vi "Add N-complement Cursors.vi"(8 "Error In":errorcluster, 9 "Cursor Mode":T1(ring), 10 "Total Cursor Number":i32=2, 11 "CrsrList in":T2) -> (0 "Error Out":errorcluster, 3 "CrsrList out":T2)   [LabVIEW 2021, in "Graphs.lvlib"]
uses:
  Graphs.lvlib
  <vilib>/Utility/miscctls.llb/LVCursorListTypeDef.ctl
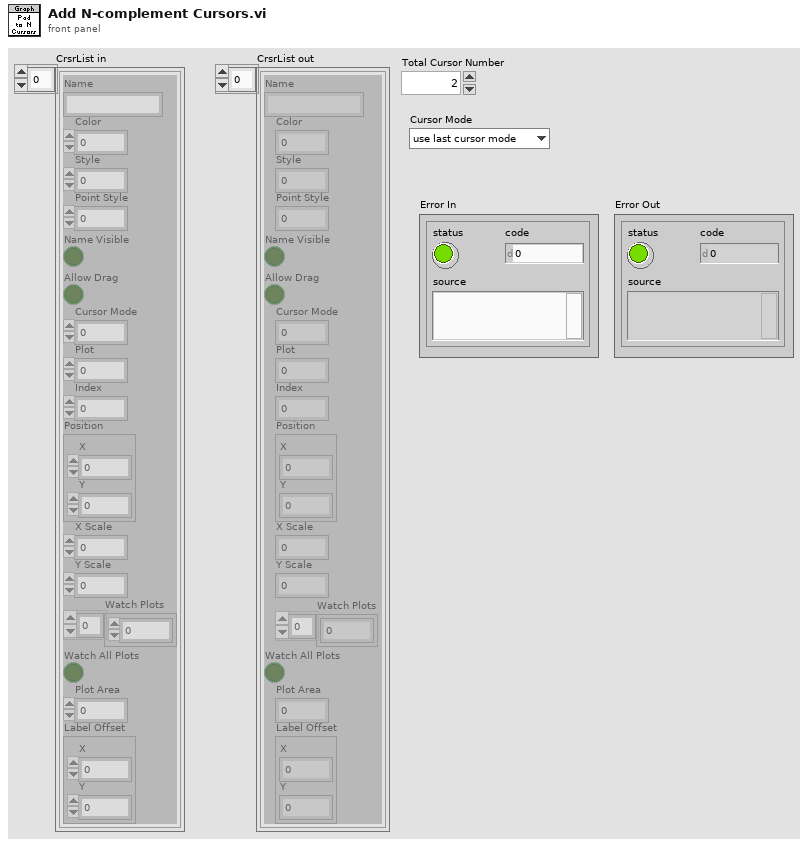
[diagram p1: front panel]
types:
  T1 = enum16{"use last cursor mode", "free", "single-plot", "multiplot"}
  T2 = typedef "LVCursorListTypeDef.ctl" = cluster{"Name":string, "Color":u32, "Style":u8, "Point Style":u8, "Name Visible":bool, "Allow Drag":bool, "Cursor Mode":u32, "Plot":i32, "Index":i32, "Position":cluster{"X":dbl, "Y":dbl}, "X Scale":u32, "Y Scale":u32, "Watch Plots":i32[], "Watch All Plots":bool, "Plot Area":i32, "Label Offset":cluster{"X":dbl, "Y":dbl}}[]
  T3 = cluster{"Name":string, "Color":u32, "Style":u8, "Point Style":u8, "Name Visible":bool, "Allow Drag":bool, "Cursor Mode":u32, "Plot":i32, "Index":i32, "Position":cluster{"X":dbl, "Y":dbl}, "X Scale":u32, "Y Scale":u32, "Watch Plots":i32[], "Watch All Plots":bool, "Plot Area":i32, "Label Offset":cluster{"X":dbl, "Y":dbl}}
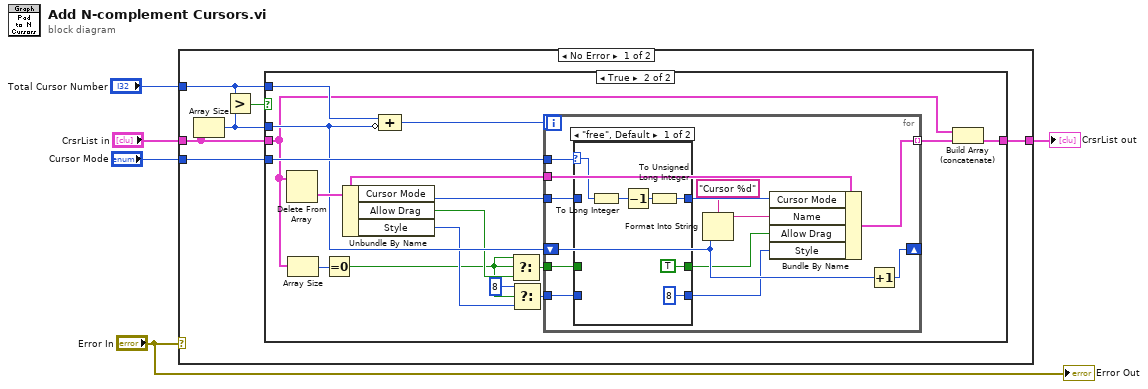
[diagram p0: block diagram]
diagram:
  n1 = case shown="No Error" "Error In" {
    tunnel: "CrsrList in" -> [w11 w51]
    tunnel: [w10 w51] -> w4
    tunnel: "Cursor Mode" -> [w9 _]
    tunnel: "Total Cursor Number" -> [w7 _]
    frame No Error {
      n2 = Array Size(array=w11) -> (size(s)=w8:i32)
      n3 = Greater?(x=w7, y=w8) -> (0:w6:bool)
      n4 = case shown="True" w6 {
        tunnel: w11 -> [w12 w13]
        tunnel: [w12 w14] -> w10
        tunnel: w8 -> [_ w23]
        tunnel: w9 -> [_ w27]
        tunnel: w7 -> [_ w24]
        frame False {
        }
        frame True {
          n5 = Delete From Array(array=w13) -> (deleted portion=w25:T3)  [unwired: 2 in, 1 out]
          n6 = Array Size(array=w13) -> (size(s)=w22:i32)
          n7 = Equal To 0?(x=w22) -> (x = 0?=w18:bool)
          n8 = Unbundle By Name(w25) -> ("Cursor Mode"=w26:u32, "Allow Drag"=w21:bool, "Style"=w19:u8)
          n9 = Compound Arithmetic op=ADD(w24, invert w23) -> (w28:i32)
          n10 = Select(t=w18, s=w18, f=w21) -> (s? t:f=w20:bool)
          n11 = Select(t=u8 8, s=w18, f=w19) -> (s? t:f=w16:u8)
          n12 = for {
            N: w28 -> [_]
            tunnel: w27 -> [w40]
            tunnel: w26 -> [w39]
            tunnel: w25 -> [w41]
            shift-right: [w37] -> _
            shift-left: w23 -> [w35]
            tunnel: w20 -> [w33]
            tunnel: w16 -> [w31]
            tunnel: [w29] -> w15 mode=indexing
            n13 = case shown="\"free\", Default" w40 {
              selector: w40 -> [w47 _]
              tunnel: w39 -> [_ w50]
              tunnel: [w44 w50] -> w38
              tunnel: w33 -> [_ w49]
              tunnel: [TRUE ("Allow Drag") w49] -> w32
              tunnel: w31 -> [_ w48]
              tunnel: [u8 8 ("Style") w48] -> w30
              frame "free", Default {
                n14 = To Long Integer(number=w47) -> (32bit integer=w45:i32)
                n15 = Decrement(x=w45) -> (x-1=w46:i32)
                n16 = To Unsigned Long Integer(number=w46) -> (unsigned 32bit integer=w44:u32)
              }
              frame "use last cursor mode" {
              }
            }
            n17 = Format Into String(format string="Cursor %d", w35) -> (resulting string=w36:string)  [unwired: 2 in, 1 out]
            n18 = Bundle By Name(cluster=w41, "Cursor Mode"=w38, "Name"=w36, "Allow Drag"=w32, "Style"=w30) -> (w29:T3)
            n19 = Increment(x=w35) -> (x+1=w37:i32)
          }
          n20 = Build Array (concatenate)(w13, w15) -> (w14:T2)
        }
      }
    }
    frame Error {
    }
  }
  "CrsrList out" <- w4
  "Error Out" <- "Error In"
